vi "move.vi"() -> ()   [LabVIEW 2013]
uses:
  <instrlib>/ZaberTSeries/Public/Utility/Response.ctl
  <vilib>/Utility/file.llb/Read From Spreadsheet File (I64).vi
  <vilib>/Utility/file.llb/Write To Spreadsheet File (I64).vi
  <instrlib>/ZaberTSeries/ZaberTSeries.lvlib
panel:
  in  "Load saved position":bool=TRUE
  in  "Save position":bool=TRUE
  in  "Path for saved position":path=path "C:/Users/lab/Dropbox/Vision software/Data/Calibration/position.txt"
  out "Current position (RV)":i32
  out "Current position (RH)":i32
  in  "Device Number (RH)":u8=4
  in  "Device Number (RV)":u8=3
  out "Current position (LH)":i32
  in  "Device Number (LH)":u8=1
  out "Current position (LV)":i32
  out "error out":errorcluster
  in  "Step Size":i32=1000
  in  "Device Number (LV)":u8=2
  in  "error in (no error)":errorcluster
  in  "VISA resource name":refnum<visa-resource-name>="COM5"
  in  "stop":bool
  # "Press space to update from saved positions."
  # "Press space after STOP to end the VI."
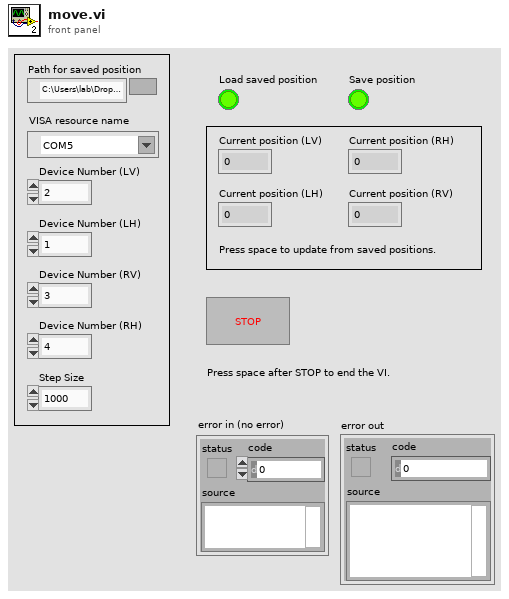
[diagram p1: front panel]
types:
  T1 = typedef "ZaberTSeries.lvlib/Response.ctl" = cluster{"Device Number":u8, "Command":u8, "Data":i32}
  T2 = cluster{"Device Number (LV)":u8, "Command":u8, "Data":i32, "Response Count":i32}
  T3 = cluster{"Device Number (LH)":u8, "Command":u8, "Data":i32, "Response Count":i32}
  T4 = cluster{"Device Number (RV)":u8, "Command":u8, "Data":i32, "Response Count":i32}
  T5 = cluster{"Device Number (RH)":u8, "Command":u8, "Data":i32, "Response Count":i32}
  T6 = enum16{"0", "1", "2", "3", "4", "5", "6", "7", "8", "9", "A", "B", "C", "D", "E", "F", "G", "H", "I", "J", "K", "L", "M", "N", "O", "P", "Q", "R", "S", "T", "U", "V", "W", "X", "Y", "Z", "F1", "F2", "F3", "F4", "F5", "F6", "F7", "F8", "F9", "F10", "F11", "F12", "F13", "F14", "F15", "ADD", "BACK", "BACKSLASH", "CAPITAL", "COMMA", "DECIMAL", "DELETE", "DIVIDE", "DOWN", "END", "EQUALS", "ESCAPE", "GRAVE (`)", "HOME", "INSERT", "LBRACKET", "LCONTROL", "LEFT", "L ALT", "LSHIFT", "LWIN", "MINUS", "MULTIPLY", "NEXT", "NUMLOCK", "NUMPAD_0", "NUMPAD_1", "NUMPAD_2", "NUMPAD_3", "NUMPAD_4", "NUMPAD_5", "NUMPAD_6", "NUMPAD_7", "NUMPAD_8", "NUMPAD_9", "PAUSE", "PERIOD", "PRIOR (PG UP)", "RBRACKET", "RCONTROL", "RETURN", "RIGHT", "R ALT", "RSHIFT", "RWIN", "SCROLL", "SEMICOLON", "SLASH", "SPACE", "SUBTRACT", "TAB", "UP", "ENTER (num pad)", "' (quote)"}
  T7 = cluster{"Device Number (LV)":u8, "Command":u8, i32, "Response Count":i32}
  T8 = cluster{"Device Number (RV)":u8, "Command":u8, i32, "Response Count":i32}
  T9 = cluster{"Device Number (LH)":u8, "Command":u8, i32, "Response Count":i32}
  T10 = cluster{"Device Number (RH)":u8, "Command":u8, i32, "Response Count":i32}
  T11 = cluster{"Device Number (LH)":u8, "Command":u8, "Step Size":i32, "Response Count":i32}
  T12 = cluster{"Device Number (RH)":u8, "Command":u8, "Step Size":i32, "Response Count":i32}
  T13 = cluster{"Device Number (LV)":u8, "Command":u8, "Step Size":i32, "Response Count":i32}
  T14 = cluster{"Device Number (RV)":u8, "Command":u8, "Step Size":i32, "Response Count":i32}
  T15 = cluster{"Response Count":i32, "Command":u8, "Response Count":i32, "Response Count":i32}
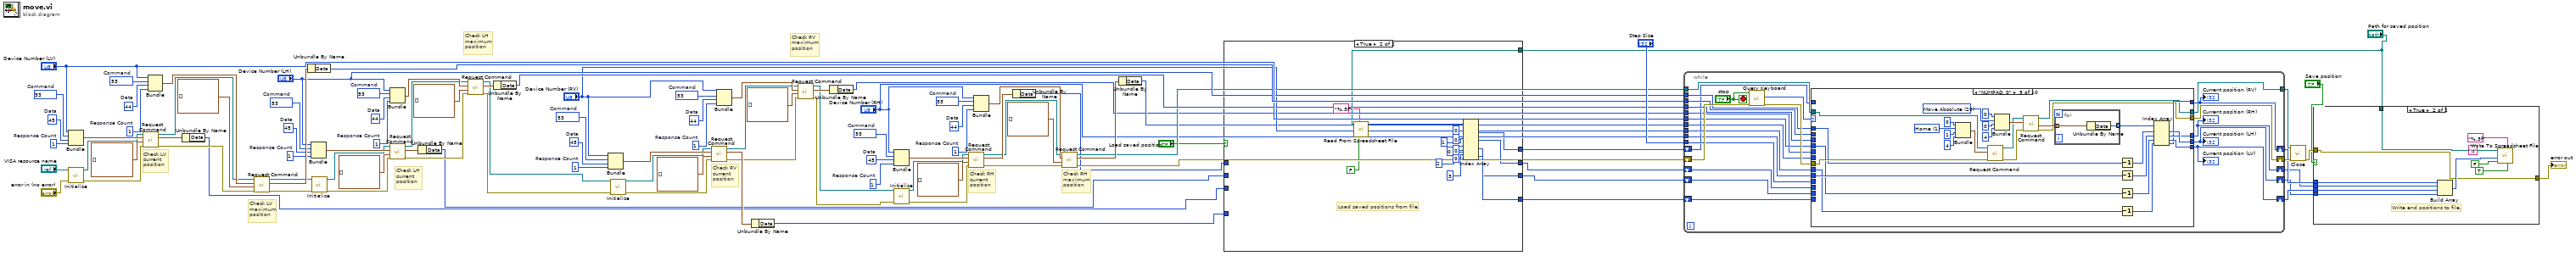
[diagram p0: block diagram]
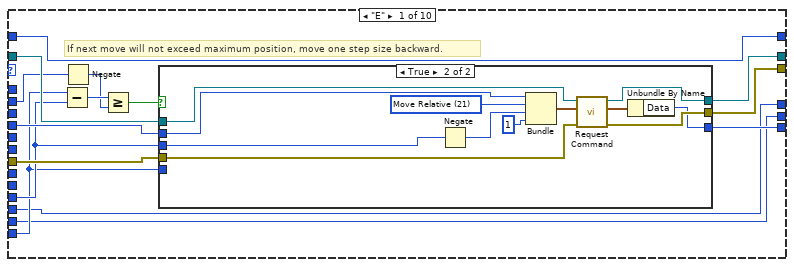
[diagram p4: hidden frame]
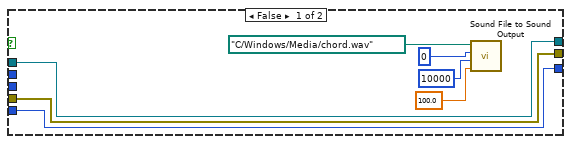
[diagram p5: hidden frame]
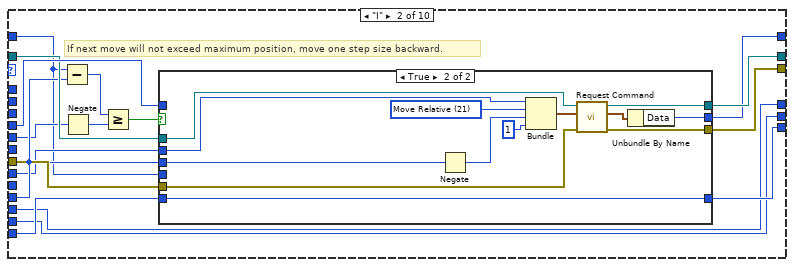
[diagram p6: hidden frame]
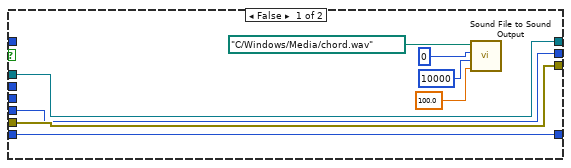
[diagram p7: hidden frame]
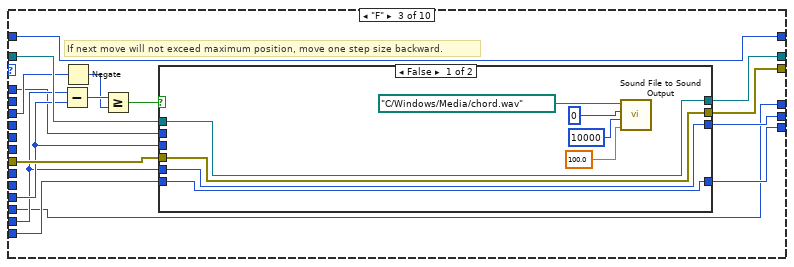
[diagram p8: hidden frame]
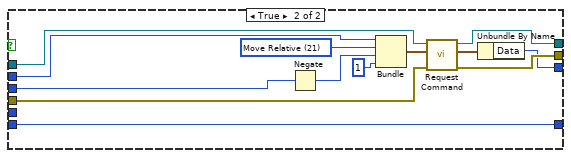
[diagram p9: hidden frame]
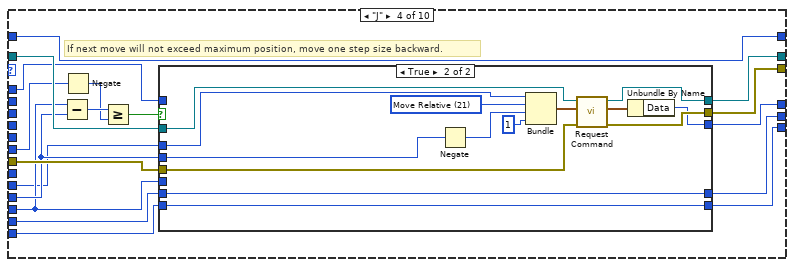
[diagram p10: hidden frame]
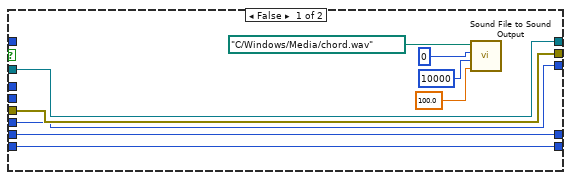
[diagram p11: hidden frame]
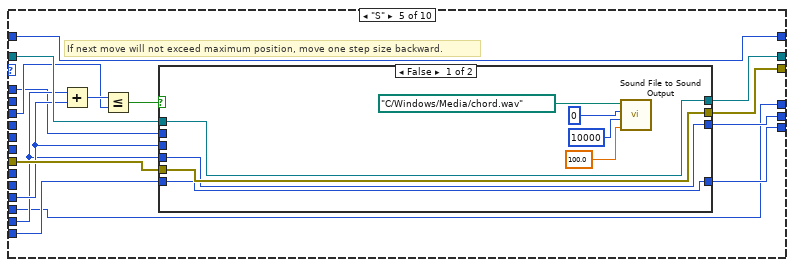
[diagram p12: hidden frame]
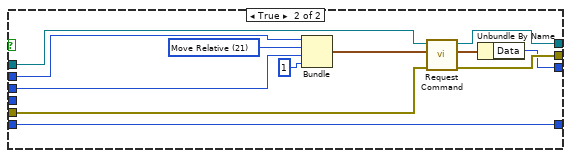
[diagram p13: hidden frame]
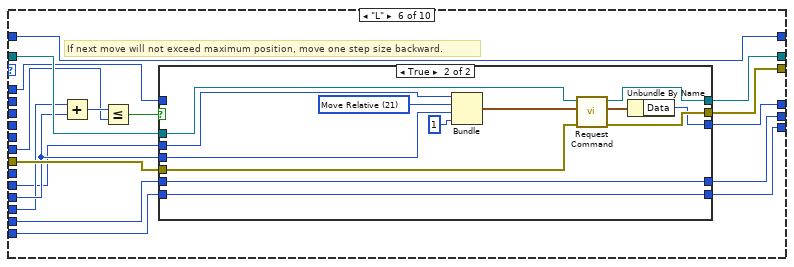
[diagram p14: hidden frame]
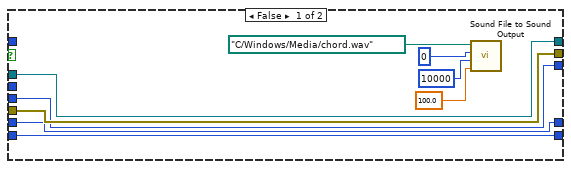
[diagram p15: hidden frame]
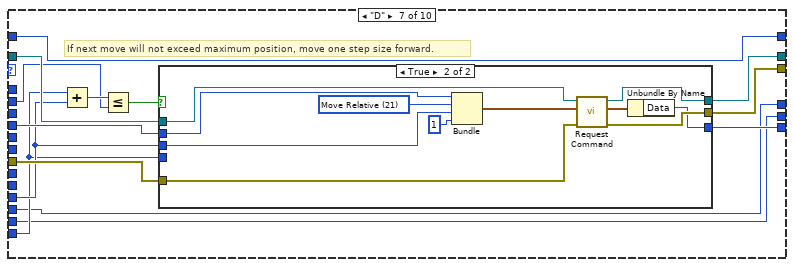
[diagram p16: hidden frame]
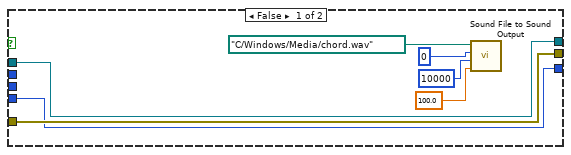
[diagram p17: hidden frame]
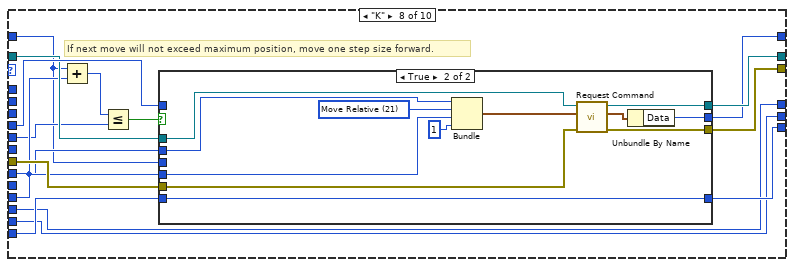
[diagram p18: hidden frame]
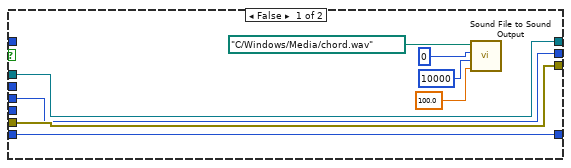
[diagram p19: hidden frame]
diagram:
  w37 = 44  # Data
  w35 = 1  # Response Count
  w38 = u8 53 items=["Echo"=55, "Home"=1, "Move Absolute"=20, "Move Relative"=21, "Move at Constant Speed"=22, "Renumber"=2, "Restore Settings"=36, "Stop"=23]  # Command
  w43 = 45  # Data
  w41 = 1  # Response Count
  w44 = u8 53 items=["Echo"=55, "Home"=1, "Move Absolute"=20, "Move Relative"=21, "Move at Constant Speed"=22, "Renumber"=2, "Restore Settings"=36, "Stop"=23]  # Command
  w53 = 44  # Data
  w51 = 1  # Response Count
  w54 = u8 53 items=["Echo"=55, "Home"=1, "Move Absolute"=20, "Move Relative"=21, "Move at Constant Speed"=22, "Renumber"=2, "Restore Settings"=36, "Stop"=23]  # Command
  w59 = 45  # Data
  w57 = 1  # Response Count
  w60 = u8 53 items=["Echo"=55, "Home"=1, "Move Absolute"=20, "Move Relative"=21, "Move at Constant Speed"=22, "Renumber"=2, "Restore Settings"=36, "Stop"=23]  # Command
  w73 = 44  # Data
  w71 = 1  # Response Count
  w74 = u8 53 items=["Echo"=55, "Home"=1, "Move Absolute"=20, "Move Relative"=21, "Move at Constant Speed"=22, "Renumber"=2, "Restore Settings"=36, "Stop"=23]  # Command
  w79 = 45  # Data
  w77 = 1  # Response Count
  w80 = u8 53 items=["Echo"=55, "Home"=1, "Move Absolute"=20, "Move Relative"=21, "Move at Constant Speed"=22, "Renumber"=2, "Restore Settings"=36, "Stop"=23]  # Command
  w92 = 44  # Data
  w90 = 1  # Response Count
  w93 = u8 53 items=["Echo"=55, "Home"=1, "Move Absolute"=20, "Move Relative"=21, "Move at Constant Speed"=22, "Renumber"=2, "Restore Settings"=36, "Stop"=23]  # Command
  w98 = 45  # Data
  w96 = 1  # Response Count
  w99 = u8 53 items=["Echo"=55, "Home"=1, "Move Absolute"=20, "Move Relative"=21, "Move at Constant Speed"=22, "Renumber"=2, "Restore Settings"=36, "Stop"=23]  # Command
  # "Check RH\nmaximum\nposition"
  # "Check RH\ncurrent \nposition"
  # "Check RV\nmaximum\nposition"
  # "Check RV\ncurrent \nposition"
  # "Check LH\nmaximum\nposition"
  # "Check LH\ncurrent \nposition"
  # "Check LV\nmaximum\nposition"
  # "Check LV\ncurrent \nposition"
  n1 = Bundle("Device Number (LV)"="Device Number (LV)", "Command"=w99, "Data"=w98, "Response Count"=w96) -> (w97:T2)  [unwired: 1 in]
  n2 = call <instrlib>:"Initialize.vi"("error in (no error)"="error in (no error)", "VISA resource name"="VISA resource name") -> ("error out"=w82:errorcluster, "VISA resource name out"=w84:refnum<visa-resource-name>)  [unwired: 7 in, 1 out]
  n3 = call <instrlib>:"Request Command.vi"("error in (no error)"=w82, "Responses in"=T1[] [], "Request"=w97, "VISA resource name"=w84) -> ("error out"=w87:errorcluster, "First Response"=w94:T1, "VISA resource name out"=w86:refnum<visa-resource-name>)  [unwired: 4 in, 1 out]
  n4 = Bundle("Device Number (LV)"="Device Number (LV)", "Command"=w93, "Data"=w92, "Response Count"=w90) -> (w91:T2)  [unwired: 1 in]
  n5 = Unbundle By Name(w94) -> ("Data"=w6:i32)
  n6 = call <instrlib>:"Request Command.vi"("error in (no error)"=w87, "Responses in"=T1[] [], "Request"=w91, "VISA resource name"=w86) -> ("error out"=w64:errorcluster, "First Response"=w88:T1, "VISA resource name out"=w63:refnum<visa-resource-name>)  [unwired: 4 in, 1 out]
  n7 = Unbundle By Name(w88) -> ("Data"=w85:i32)
  n8 = Bundle("Device Number (LH)"="Device Number (LH)", "Command"=w80, "Data"=w79, "Response Count"=w77) -> (w78:T3)  [unwired: 1 in]
  n9 = call <instrlib>:"Initialize.vi"("error in (no error)"=w64, "VISA resource name"=w63) -> ("error out"=w65:errorcluster, "VISA resource name out"=w66:refnum<visa-resource-name>)  [unwired: 7 in, 1 out]
  n10 = Bundle("Device Number (LH)"="Device Number (LH)", "Command"=w74, "Data"=w73, "Response Count"=w71) -> (w72:T3)  [unwired: 1 in]
  n11 = call <instrlib>:"Request Command.vi"("error in (no error)"=w65, "Responses in"=T1[] [], "Request"=w78, "VISA resource name"=w66) -> ("error out"=w68:errorcluster, "First Response"=w75:T1, "VISA resource name out"=w67:refnum<visa-resource-name>)  [unwired: 4 in, 1 out]
  n12 = Unbundle By Name(w75) -> ("Data"=w4:i32)
  n13 = call <instrlib>:"Request Command.vi"("error in (no error)"=w68, "Responses in"=T1[] [], "Request"=w72, "VISA resource name"=w67) -> ("error out"=w26:errorcluster, "First Response"=w69:T1, "VISA resource name out"=w25:refnum<visa-resource-name>)  [unwired: 4 in, 1 out]
  n14 = Unbundle By Name(w69) -> ("Data"=w62:i32)
  n15 = Bundle("Device Number (RV)"="Device Number (RV)", "Command"=w60, "Data"=w59, "Response Count"=w57) -> (w58:T4)  [unwired: 1 in]
  n16 = call <instrlib>:"Initialize.vi"("error in (no error)"=w26, "VISA resource name"=w25) -> ("error out"=w45:errorcluster, "VISA resource name out"=w46:refnum<visa-resource-name>)  [unwired: 7 in, 1 out]
  n17 = call <instrlib>:"Request Command.vi"("error in (no error)"=w45, "Responses in"=T1[] [], "Request"=w58, "VISA resource name"=w46) -> ("error out"=w48:errorcluster, "First Response"=w55:T1, "VISA resource name out"=w47:refnum<visa-resource-name>)  [unwired: 4 in, 1 out]
  n18 = Bundle("Device Number (RV)"="Device Number (RV)", "Command"=w54, "Data"=w53, "Response Count"=w51) -> (w52:T4)  [unwired: 1 in]
  n19 = Unbundle By Name(w55) -> ("Data"=w8:i32)
  n20 = call <instrlib>:"Request Command.vi"("error in (no error)"=w48, "Responses in"=T1[] [], "Request"=w52, "VISA resource name"=w47) -> ("error out"=w28:errorcluster, "First Response"=w49:T1, "VISA resource name out"=w27:refnum<visa-resource-name>)  [unwired: 4 in, 1 out]
  n21 = Unbundle By Name(w49) -> ("Data"=w18:i32)
  n22 = Bundle("Device Number (RH)"="Device Number (RH)", "Command"=w44, "Data"=w43, "Response Count"=w41) -> (w42:T5)  [unwired: 1 in]
  n23 = call <instrlib>:"Initialize.vi"("error in (no error)"=w28, "VISA resource name"=w27) -> ("error out"=w29:errorcluster, "VISA resource name out"=w30:refnum<visa-resource-name>)  [unwired: 7 in, 1 out]
  n24 = call <instrlib>:"Request Command.vi"("error in (no error)"=w29, "Responses in"=T1[] [], "Request"=w42, "VISA resource name"=w30) -> ("error out"=w32:errorcluster, "First Response"=w39:T1, "VISA resource name out"=w31:refnum<visa-resource-name>)  [unwired: 4 in, 1 out]
  n25 = Bundle("Device Number (RH)"="Device Number (RH)", "Command"=w38, "Data"=w37, "Response Count"=w35) -> (w36:T5)  [unwired: 1 in]
  n26 = Unbundle By Name(w39) -> ("Data"=w2:i32)
  n27 = call <instrlib>:"Request Command.vi"("error in (no error)"=w32, "Responses in"=T1[] [], "Request"=w36, "VISA resource name"=w31) -> ("error out"=w21:errorcluster, "First Response"=w33:T1, "VISA resource name out"=w24:refnum<visa-resource-name>)  [unwired: 4 in, 1 out]
  n28 = Unbundle By Name(w33) -> ("Data"=w20:i32)
  n29 = case shown="True" "Load saved position" {
    tunnel: "Path for saved position" -> [_ w122]
    tunnel: w8 -> [w106 _]
    tunnel: [w106 w111] -> w7
    tunnel: w6 -> [w105 _]
    tunnel: [w105 w109] -> w5
    tunnel: [w104 w108] -> w3
    tunnel: w4 -> [w104 _]
    tunnel: [w103 w110] -> w1
    tunnel: w2 -> [w103 _]
    frame False {
    }
    frame True {
      # "Load saved positions from file."
      n30 = call-poly <vilib>:"Read From Spreadsheet File.vi"("transpose (no:F)"=FALSE, "format (%d)"="%.3f" ("format (%.3f)"), "file path (dialog if empty)"=w122) -> ("all rows"=w107:i64[][])  [unwired: 4 in, 4 out]
      n31 = Index Array(array=w107, index (row) #1=0 ("index"), index (col) #1=0 ("disabled index (col)"), index (row) #2=1 ("index"), index (col) #2=0 ("disabled index (col)"), index (row) #3=2 ("index"), index (col) #3=0 ("disabled index (col)"), index (row) #4=3 ("index"), index (col) #4=0 ("disabled index (col)")) -> (element #1=w111:i64, element #2=w110:i64, element #3=w109:i64, element #4=w108:i64)
    }
  }
  n32 = while {
    shift-right: [w144] -> w100
    shift-left: w21 -> [w146]
    tunnel: "Step Size" -> [w142]
    tunnel: "Device Number (LV)" -> [w141]
    tunnel: w24 -> [w140]
    tunnel: [w139] -> w19
    shift-right: [w138] -> w15
    shift-left: w5 -> [w132]
    tunnel: w85 -> [w137]
    tunnel: w62 -> [w133]
    shift-right: [w135] -> w14
    shift-left: w3 -> [w134]
    tunnel: "Device Number (LH)" -> [w131]
    tunnel: "Device Number (RH)" -> [w128]
    tunnel: "Device Number (RV)" -> [w130]
    tunnel: w20 -> [w127]
    shift-right: [w126] -> w16
    shift-left: w1 -> [w125]
    tunnel: w18 -> [w124]
    shift-right: [w123] -> w17
    shift-left: w7 -> [w129]
    stop <- "stop" stop-if-true
    n33 = call "Query Keyboard.vi"("error in (no error)"=w146, "Stop?"="stop") -> ("error out"=w145:errorcluster, "element"=w143:T6)  [unwired: 8 in]
    n34 = case shown="\"NUMPAD_0\"" w143 {
      tunnel: w145 -> [w157 w193 w231 w270 w308 w345 w380 w414 w464 w476]
      tunnel: [w160 w196 w234 w273 w311 w348 w383 w417 w441 w476] -> w144
      tunnel: w140 -> [w159 w195 w233 w272 w310 w347 w382 w416 w465 w475]
      tunnel: w142 -> [w155 w191 w229 w268 w306 w343 w378 w412 _ _]
      tunnel: w141 -> [w161 w197 _ _ _ _ w384 w418 w453 _]
      tunnel: [w158 w194 w232 w271 w309 w346 w381 w415 w439 w475] -> w139
      tunnel: [w156 w192 w230 w269 w307 w344 w379 w413 w452 w474] -> w138
      tunnel: w132 -> [w150 w187 w225 w264 w303 w340 w376 w410 _ w474]
      tunnel: w137 -> [w153 _ _ _ _ _ w374 _ _ _]
      tunnel: [w149 w186 w224 w263 w302 w339 w373 w408 w460 w473] -> w135
      tunnel: w134 -> [w149 w186 w222 w259 w301 w337 w373 w408 _ w473]
      tunnel: w133 -> [_ _ w223 _ w300 _ _ _ _ _]
      tunnel: w131 -> [_ _ w221 w262 w299 w338 _ _ w459 _]
      tunnel: w130 -> [_ w182 _ _ _ _ _ w406 w450 _]
      tunnel: w129 -> [w147 w181 w219 w256 w297 w332 w371 w403 _ w471]
      tunnel: w128 -> [_ _ _ w257 _ w333 _ _ w456 _]
      tunnel: w127 -> [_ _ _ w260 _ w334 _ _ _ _]
      tunnel: [w148 w185 w220 w261 w298 w336 w372 w407 w455 w472] -> w126
      tunnel: w125 -> [w148 w185 w220 w258 w298 w335 w372 w407 _ w472]
      tunnel: w124 -> [_ w184 _ _ _ _ _ w405 _ _]
      tunnel: [w147 w183 w219 w256 w297 w332 w371 w404 w449 w471] -> w123
      frame "E" {
        # "If next move will not exceed maximum position, move one step size backward."
        n35 = Subtract(x=w150, y=w155) -> (x-y=w154:i64)
        n36 = Negate(x=w153) -> (-x=w152:i32)
        n37 = Greater Or Equal?(x=w154, y=w152) -> (x >= y?=w151:bool)
        n38 = case shown="True" w151 {
          tunnel: w155 -> [_ w176]
          tunnel: w161 -> [_ w175]
          tunnel: w159 -> [w162 w174]
          tunnel: [w168 w173] -> w160
          tunnel: [w162 w172] -> w158
          tunnel: w157 -> [w168 w169]
          tunnel: [w167 w170] -> w156
          tunnel: w150 -> [w167 _]
          frame False {
            n39 = call "Sound File to Sound Output.vi"("Volume"=100.0, "Number of Samples/Iteration"=10000, "Device ID"=u32 0, "File Path"=path "C:/Windows/Media/chord.wav") -> ()
          }
          frame True {
            w177 = u8 21 items=["Echo"=55, "Home"=1, "Move Absolute"=20, "Move Relative"=21, "Move at Constant Speed"=22, "Renumber"=2, "Restore Settings"=36, "Stop"=23] ("Command")
            n40 = Negate(x=w176) -> (-x=w180:i32)
            n41 = Bundle("Device Number (LV)"=w175, "Command"=w177, w180, "Response Count"=1) -> (w179:T7)  [unwired: 1 in]
            n42 = call <instrlib>:"Request Command.vi"("error in (no error)"=w169, "Request"=w179, "VISA resource name"=w174) -> ("error out"=w173:errorcluster, "First Response"=w171:T1, "VISA resource name out"=w172:refnum<visa-resource-name>)  [unwired: 5 in, 1 out]
            n43 = Unbundle By Name(w171) -> ("Data"=w170:i32)
          }
        }
      }
      frame "I" {
        # "If next move will not exceed maximum position, move one step size backward."
        n44 = Subtract(x=w181, y=w191) -> (x-y=w190:i64)
        n45 = Negate(x=w184) -> (-x=w189:i32)
        n46 = Greater Or Equal?(x=w190, y=w189) -> (x >= y?=w188:bool)
        n47 = case shown="True" w188 {
          tunnel: w191 -> [_ w214]
          tunnel: w197 -> [_ _]
          tunnel: w195 -> [w199 w213]
          tunnel: [w205 w212] -> w196
          tunnel: [w199 w211] -> w194
          tunnel: w193 -> [w205 w209]
          tunnel: [w204 w208] -> w192
          tunnel: w187 -> [w204 w208]
          tunnel: [w198 w207] -> w183
          tunnel: w182 -> [_ w206]
          tunnel: w181 -> [w198 _]
          frame False {
            n48 = call "Sound File to Sound Output.vi"("Volume"=100.0, "Number of Samples/Iteration"=10000, "Device ID"=u32 0, "File Path"=path "C:/Windows/Media/chord.wav") -> ()
          }
          frame True {
            w215 = u8 21 items=["Echo"=55, "Home"=1, "Move Absolute"=20, "Move Relative"=21, "Move at Constant Speed"=22, "Renumber"=2, "Restore Settings"=36, "Stop"=23] ("Command")
            n49 = Negate(x=w214) -> (-x=w218:i32)
            n50 = Bundle("Device Number (RV)"=w206, "Command"=w215, w218, "Response Count"=1) -> (w217:T8)  [unwired: 1 in]
            n51 = call <instrlib>:"Request Command.vi"("error in (no error)"=w209, "Request"=w217, "VISA resource name"=w213) -> ("error out"=w212:errorcluster, "First Response"=w210:T1, "VISA resource name out"=w211:refnum<visa-resource-name>)  [unwired: 5 in, 1 out]
            n52 = Unbundle By Name(w210) -> ("Data"=w207:i32)
          }
        }
      }
      frame "F" {
        # "If next move will not exceed maximum position, move one step size backward."
        n53 = Subtract(x=w222, y=w229) -> (x-y=w228:i64)
        n54 = Negate(x=w223) -> (-x=w227:i32)
        n55 = Greater Or Equal?(x=w228, y=w227) -> (x >= y?=w226:bool)
        n56 = case shown="False" w226 {
          tunnel: w229 -> [_ w251]
          tunnel: w221 -> [_ w250]
          tunnel: w233 -> [w236 w249]
          tunnel: [w242 w248] -> w234
          tunnel: [w236 w247] -> w232
          tunnel: w231 -> [w242 w245]
          tunnel: [w241 w244] -> w230
          tunnel: w225 -> [w241 w244]
          tunnel: [w235 w243] -> w224
          tunnel: w222 -> [w235 _]
          frame False {
            n57 = call "Sound File to Sound Output.vi"("Volume"=100.0, "Number of Samples/Iteration"=10000, "Device ID"=u32 0, "File Path"=path "C:/Windows/Media/chord.wav") -> ()
          }
          frame True {
            w252 = u8 21 items=["Echo"=55, "Home"=1, "Move Absolute"=20, "Move Relative"=21, "Move at Constant Speed"=22, "Renumber"=2, "Restore Settings"=36, "Stop"=23] ("Command")
            n58 = Negate(x=w251) -> (-x=w255:i32)
            n59 = Bundle("Device Number (LH)"=w250, "Command"=w252, w255, "Response Count"=1) -> (w254:T9)  [unwired: 1 in]
            n60 = call <instrlib>:"Request Command.vi"("error in (no error)"=w245, "Request"=w254, "VISA resource name"=w249) -> ("error out"=w248:errorcluster, "First Response"=w246:T1, "VISA resource name out"=w247:refnum<visa-resource-name>)  [unwired: 5 in, 1 out]
            n61 = Unbundle By Name(w246) -> ("Data"=w243:i32)
          }
        }
      }
      frame "J" {
        # "If next move will not exceed maximum position, move one step size backward."
        n62 = Subtract(x=w258, y=w268) -> (x-y=w267:i64)
        n63 = Negate(x=w260) -> (-x=w266:i32)
        n64 = Greater Or Equal?(x=w267, y=w266) -> (x >= y?=w265:bool)
        n65 = case shown="True" w265 {
          tunnel: w268 -> [_ w292]
          tunnel: w262 -> [_ _]
          tunnel: w272 -> [w276 w291]
          tunnel: [w282 w290] -> w273
          tunnel: [w276 w289] -> w271
          tunnel: w270 -> [w282 w287]
          tunnel: [w281 w286] -> w269
          tunnel: w264 -> [w281 w286]
          tunnel: [w275 w285] -> w263
          tunnel: w259 -> [w275 w285]
          tunnel: [w274 w284] -> w261
          tunnel: w258 -> [w274 _]
          tunnel: w257 -> [_ w283]
          frame False {
            n66 = call "Sound File to Sound Output.vi"("Volume"=100.0, "Number of Samples/Iteration"=10000, "Device ID"=u32 0, "File Path"=path "C:/Windows/Media/chord.wav") -> ()
          }
          frame True {
            w293 = u8 21 items=["Echo"=55, "Home"=1, "Move Absolute"=20, "Move Relative"=21, "Move at Constant Speed"=22, "Renumber"=2, "Restore Settings"=36, "Stop"=23] ("Command")
            n67 = Negate(x=w292) -> (-x=w296:i32)
            n68 = Bundle("Device Number (RH)"=w283, "Command"=w293, w296, "Response Count"=1) -> (w295:T10)  [unwired: 1 in]
            n69 = call <instrlib>:"Request Command.vi"("error in (no error)"=w287, "Request"=w295, "VISA resource name"=w291) -> ("error out"=w290:errorcluster, "First Response"=w288:T1, "VISA resource name out"=w289:refnum<visa-resource-name>)  [unwired: 5 in, 1 out]
            n70 = Unbundle By Name(w288) -> ("Data"=w284:i32)
          }
        }
      }
      frame "S" {
        # "If next move will not exceed maximum position, move one step size backward."
        n71 = Add(x=w301, y=w306) -> (x+y=w305:i64)
        n72 = Less Or Equal?(x=w305, y=w300) -> (x <= y?=w304:bool)
        n73 = case shown="False" w304 {
          tunnel: w306 -> [_ w320]
          tunnel: w299 -> [_ w328]
          tunnel: w310 -> [w313 w327]
          tunnel: [w319 w326] -> w311
          tunnel: [w313 w325] -> w309
          tunnel: w308 -> [w319 w323]
          tunnel: [w318 w322] -> w307
          tunnel: w303 -> [w318 w322]
          tunnel: [w312 w321] -> w302
          tunnel: w301 -> [w312 _]
          frame False {
            n74 = call "Sound File to Sound Output.vi"("Volume"=100.0, "Number of Samples/Iteration"=10000, "Device ID"=u32 0, "File Path"=path "C:/Windows/Media/chord.wav") -> ()
          }
          frame True {
            w329 = u8 21 items=["Echo"=55, "Home"=1, "Move Absolute"=20, "Move Relative"=21, "Move at Constant Speed"=22, "Renumber"=2, "Restore Settings"=36, "Stop"=23] ("Command")
            n75 = Bundle("Device Number (LH)"=w328, "Command"=w329, "Step Size"=w320, "Response Count"=1) -> (w331:T11)  [unwired: 1 in]
            n76 = call <instrlib>:"Request Command.vi"("error in (no error)"=w323, "Request"=w331, "VISA resource name"=w327) -> ("error out"=w326:errorcluster, "First Response"=w324:T1, "VISA resource name out"=w325:refnum<visa-resource-name>)  [unwired: 5 in, 1 out]
            n77 = Unbundle By Name(w324) -> ("Data"=w321:i32)
          }
        }
      }
      frame "L" {
        # "If next move will not exceed maximum position, move one step size backward."
        n78 = Add(x=w335, y=w343) -> (x+y=w342:i64)
        n79 = Less Or Equal?(x=w342, y=w334) -> (x <= y?=w341:bool)
        n80 = case shown="True" w341 {
          tunnel: w343 -> [w349 w361]
          tunnel: w338 -> [_ _]
          tunnel: w347 -> [w351 w367]
          tunnel: [w357 w366] -> w348
          tunnel: [w351 w365] -> w346
          tunnel: w345 -> [w357 w363]
          tunnel: [w356 w362] -> w344
          tunnel: w340 -> [w356 w362]
          tunnel: [w350 w360] -> w339
          tunnel: w337 -> [w350 w360]
          tunnel: [w349 w359] -> w336
          tunnel: w333 -> [_ w358]
          frame False {
            n81 = call "Sound File to Sound Output.vi"("Volume"=100.0, "Number of Samples/Iteration"=10000, "Device ID"=u32 0, "File Path"=path "C:/Windows/Media/chord.wav") -> ()
          }
          frame True {
            w368 = u8 21 items=["Echo"=55, "Home"=1, "Move Absolute"=20, "Move Relative"=21, "Move at Constant Speed"=22, "Renumber"=2, "Restore Settings"=36, "Stop"=23] ("Command")
            n82 = Bundle("Device Number (RH)"=w358, "Command"=w368, "Step Size"=w361, "Response Count"=1) -> (w370:T12)  [unwired: 1 in]
            n83 = call <instrlib>:"Request Command.vi"("error in (no error)"=w363, "Request"=w370, "VISA resource name"=w367) -> ("error out"=w366:errorcluster, "First Response"=w364:T1, "VISA resource name out"=w365:refnum<visa-resource-name>)  [unwired: 5 in, 1 out]
            n84 = Unbundle By Name(w364) -> ("Data"=w359:i32)
          }
        }
      }
      frame "D" {
        # "If next move will not exceed maximum position, move one step size forward."
        n85 = Add(x=w376, y=w378) -> (x+y=w375:i64)
        n86 = Less Or Equal?(x=w375, y=w374) -> (x <= y?=w377:bool)
        n87 = case shown="True" w377 {
          tunnel: w378 -> [_ w393]
          tunnel: w384 -> [_ w399]
          tunnel: w382 -> [w385 w398]
          tunnel: [w387 w397] -> w383
          tunnel: [w385 w396] -> w381
          tunnel: w380 -> [w387 w392]
          tunnel: [w386 w394] -> w379
          tunnel: w376 -> [w386 _]
          frame False {
            n88 = call "Sound File to Sound Output.vi"("Volume"=100.0, "Number of Samples/Iteration"=10000, "Device ID"=u32 0, "File Path"=path "C:/Windows/Media/chord.wav") -> ()
          }
          frame True {
            w400 = u8 21 items=["Echo"=55, "Home"=1, "Move Absolute"=20, "Move Relative"=21, "Move at Constant Speed"=22, "Renumber"=2, "Restore Settings"=36, "Stop"=23] ("Command")
            n89 = Bundle("Device Number (LV)"=w399, "Command"=w400, "Step Size"=w393, "Response Count"=1) -> (w402:T13)  [unwired: 1 in]
            n90 = call <instrlib>:"Request Command.vi"("error in (no error)"=w392, "Request"=w402, "VISA resource name"=w398) -> ("error out"=w397:errorcluster, "First Response"=w395:T1, "VISA resource name out"=w396:refnum<visa-resource-name>)  [unwired: 5 in, 1 out]
            n91 = Unbundle By Name(w395) -> ("Data"=w394:i32)
          }
        }
      }
      frame "K" {
        # "If next move will not exceed maximum position, move one step size forward."
        n92 = Add(x=w403, y=w412) -> (x+y=w409:i64)
        n93 = Less Or Equal?(x=w409, y=w405) -> (x <= y?=w411:bool)
        n94 = case shown="True" w411 {
          tunnel: w412 -> [_ w431]
          tunnel: w418 -> [_ _]
          tunnel: w416 -> [w420 w435]
          tunnel: [w422 w434] -> w417
          tunnel: [w420 w433] -> w415
          tunnel: w414 -> [w422 w430]
          tunnel: [w421 w427] -> w413
          tunnel: w410 -> [w421 w427]
          tunnel: w406 -> [_ w429]
          tunnel: [w419 w428] -> w404
          tunnel: w403 -> [w419 _]
          frame False {
            n95 = call "Sound File to Sound Output.vi"("Volume"=100.0, "Number of Samples/Iteration"=10000, "Device ID"=u32 0, "File Path"=path "C:/Windows/Media/chord.wav") -> ()
          }
          frame True {
            w436 = u8 21 items=["Echo"=55, "Home"=1, "Move Absolute"=20, "Move Relative"=21, "Move at Constant Speed"=22, "Renumber"=2, "Restore Settings"=36, "Stop"=23] ("Command")
            n96 = Bundle("Device Number (RV)"=w429, "Command"=w436, "Step Size"=w431, "Response Count"=1) -> (w438:T14)  [unwired: 1 in]
            n97 = call <instrlib>:"Request Command.vi"("error in (no error)"=w430, "Request"=w438, "VISA resource name"=w435) -> ("error out"=w434:errorcluster, "First Response"=w432:T1, "VISA resource name out"=w433:refnum<visa-resource-name>)  [unwired: 5 in, 1 out]
            n98 = Unbundle By Name(w432) -> ("Data"=w428:i32)
          }
        }
      }
      frame "NUMPAD_0" {
        w446 = u8 20 items=["Echo"=55, "Home"=1, "Move Absolute"=20, "Move Relative"=21, "Move at Constant Speed"=22, "Renumber"=2, "Restore Settings"=36, "Stop"=23] ("Command")
        w466 = u8 1 items=["Echo"=55, "Home"=1, "Move Absolute"=20, "Move Relative"=21, "Move at Constant Speed"=22, "Renumber"=2, "Restore Settings"=36, "Stop"=23] ("Command")
        n99 = Bundle("Response Count"=0, "Command"=w466, "Response Count"=1, "Response Count"=4) -> (w468:T15)  [unwired: 1 in]
        n100 = call <instrlib>:"Request Command.vi"("error in (no error)"=w464, "Request"=w468, "VISA resource name"=w465) -> ("error out"=w442:errorcluster, "VISA resource name out"=w440:refnum<visa-resource-name>)  [unwired: 5 in, 2 out]
        n101 = Bundle("Response Count"=0, "Command"=w446, "Response Count"=0, "Response Count"=4) -> (w448:T15)  [unwired: 1 in]
        n102 = call <instrlib>:"Request Command.vi"("error in (no error)"=w442, "Request"=w448, "VISA resource name"=w440) -> ("error out"=w441:errorcluster, "Responses out"=w443:T1[], "VISA resource name out"=w439:refnum<visa-resource-name>)  [unwired: 5 in, 1 out]
        n103 = for {
          tunnel: w443 -> [w470] mode=indexing
          tunnel: [w469] -> w461 mode=indexing
          n104 = Unbundle By Name(w470) -> ("Data"=w469:i32)
        }
        n105 = Decrement(x=w459) -> (x-1=w458:u8)
        n106 = Decrement(x=w456) -> (x-1=w457:u8)
        n107 = Decrement(x=w453) -> (x-1=w454:u8)
        n108 = Decrement(x=w450) -> (x-1=w451:u8)
        n109 = Index Array(array=w461, index #1=w458, index #2=w457, index #3=w454, index #4=w451) -> (element #1=w460:i32, element #2=w455:i32, element #3=w452:i32, element #4=w449:i32)
      }
      frame "SPACE", Default {
      }
    }
    "Current position (LV)" <- w138
    "Current position (LH)" <- w135
    "Current position (RH)" <- w126
    "Current position (RV)" <- w123
  }
  n110 = call <instrlib>:"Close.vi"("error in (no error)"=w100, "VISA resource name"=w19) -> ("error out"=w13:errorcluster)  [unwired: 8 in, 1 out]
  n111 = case shown="True" "Save position" {
    tunnel: w17 -> [_ w488]
    tunnel: w16 -> [_ w487]
    tunnel: w15 -> [_ w486]
    tunnel: w14 -> [_ w485]
    tunnel: "Path for saved position" -> [_ w484]
    tunnel: w13 -> [w477 w478]
    tunnel: [w477 w478] -> w12
    frame False {
    }
    frame True {
      # "Write end positions to file."
      n112 = Build Array(w488, w487, w486, w485) -> (w479:i64[])
      n113 = call-poly <vilib>:"Write To Spreadsheet File.vi"("delimiter (\\t)"="\t" ("delimiter (\\t)"), "transpose? (no:F)"=TRUE, "format (%d)"="%.3f" ("format (%.3f)"), "append to file? (new file:F)"=FALSE, "1D data"=w479, "file path (dialog if empty)"=w484) -> ()  [unwired: 2 in, 1 out]
    }
  }
  "error out" <- w12
